vi "Actor Core.vi"(8 "error in":errorcluster, 11 "Nested in":refnum<class "GUI_Actor.lvclass">) -> (0 "error out":errorcluster, 3 "Actor out":refnum<class "Actor.lvclass">)   [LabVIEW 2019, in "GUI_Actor.lvlib" / "GUI_Actor.lvclass"]
doc: "(<B>Filename</B>: Actor Framework.lvlib:Actor.lvclass:Actor Core.vi)\n\nReceives messages to the actor, reacts to them, and initiates any error handling that may shut the actor down.\n\nDescendant classes may override this VI to append parallel tasks for the actor to complete while it handles messages. Overrides use the Call Parent Method node."
uses:
  GUI_Actor.lvclass
  C:/Program Files/National Instruments/LabVIEW 2019/vi.lib/ActorFramework/Actor/Actor.lvclass
  <vilib>/ActorFramework/Actor/Actor.lvclass
  Signal_Gen/Signal_Gen/Signal_Gen.lvclass
  Logging_txt/Logging_txt/Logging_txt.lvclass
  GUI_Actor.lvclass/GUI_Actor.ctl
  <vilib>/ActorFramework/Actor/Actor.lvclass/Actor.ctl
  <vilib>/ActorFramework/Message Enqueuer/Message Enqueuer.lvclass/Message Enqueuer.ctl
  GUI_Actor Messages/Start_Stop Msg/Start_Stop Msg.lvclass/Start_Stop Msg.ctl
  GUI_Actor Messages/Save_enable Msg/Save_enable Msg.lvclass/Save_enable Msg.ctl
  GUI_Actor Messages/File_path Msg/File_path Msg.lvclass/File_path Msg.ctl
  <vilib>/ActorFramework/Message Enqueuer/Init from Existing Queue.vi
  <vilib>/ActorFramework/Message Enqueuer/Enqueue.vi
  <vilib>/ActorFramework/Stop Msg/Stop Msg.lvclass
  C:/Program Files/National Instruments/LabVIEW 2019/vi.lib/ActorFramework/Message/Message.lvclass
  GUI_Actor Messages/Start_Stop Msg/Start_Stop Msg.lvclass
  GUI_Actor Messages/Save_enable Msg/Save_enable Msg.lvclass
  GUI_Actor Messages/File_path Msg/File_path Msg.lvclass
  <vilib>/ActorFramework/Message Priority Queue/Priority Enqueue.vi
  <vilib>/ActorFramework/Message Enqueuer/Message Enqueuer.lvclass
panel:
  out "Grafica":waveform(dbl)(graph)
  in  "Formato":enum16{"TXT", "TDMS"}(ring)
  in  "Amplitud":dbl
  in  "Frecuencia":dbl
  in  "Tipo de señal":enum16{"Senoidal", "Cuadrada", "Triangular"}(ring)
  in  "Stop":bool
  in  "Start":bool
  in  "Save":bool
  in  "Direccion":path
  in  "Exit":bool
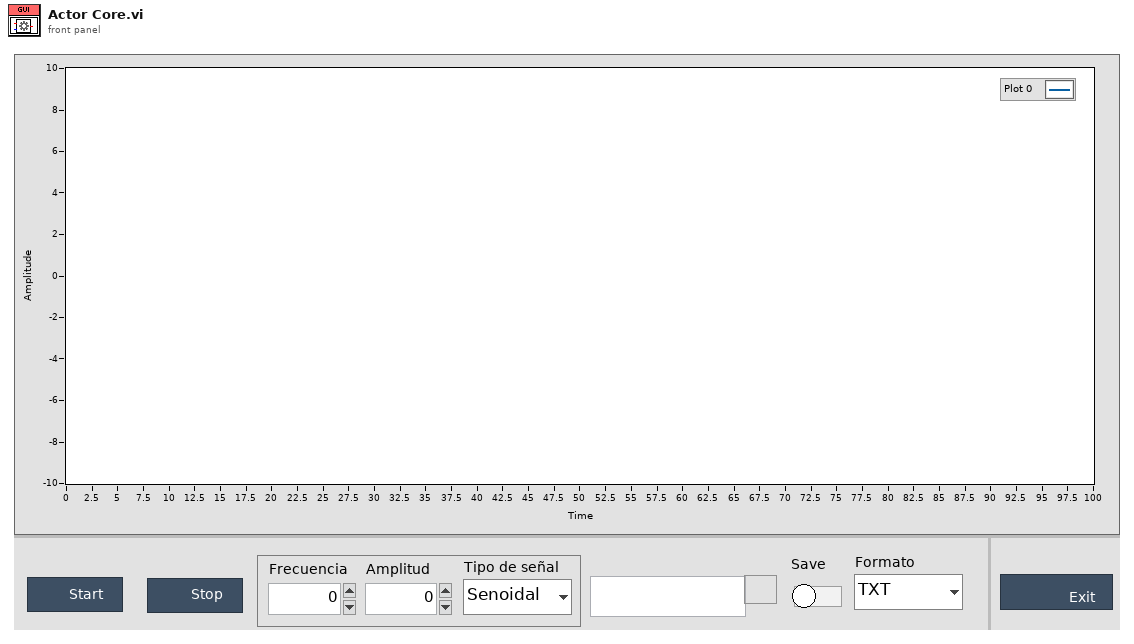
[diagram p1: front panel]
types:
  T1 = cluster{"Stop":refnum<user-event>, "Grafica":refnum<user-event>}
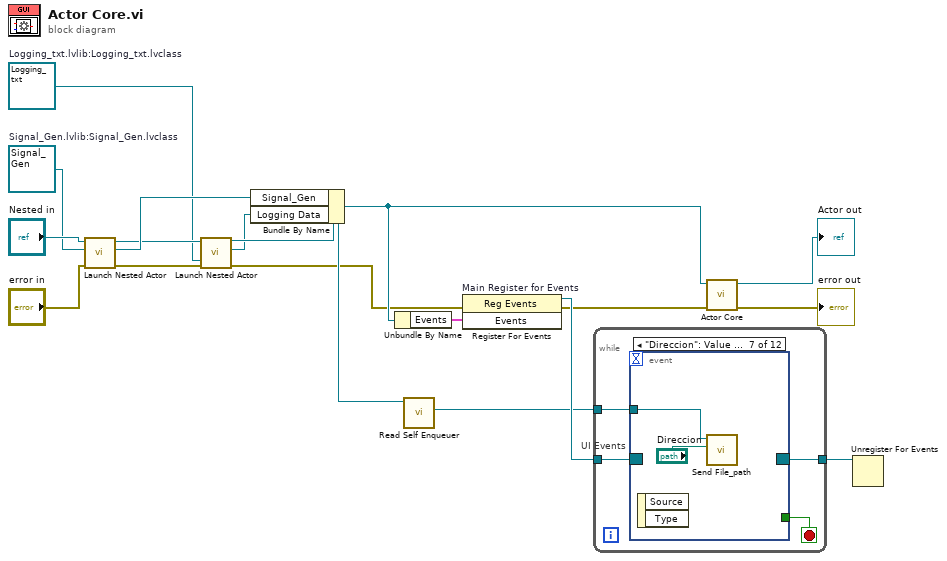
[diagram p0: block diagram]
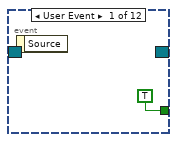
[diagram p2: hidden frame]
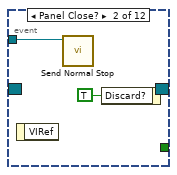
[diagram p3: hidden frame]
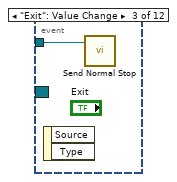
[diagram p4: hidden frame]
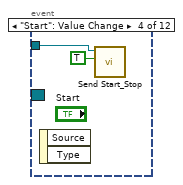
[diagram p5: hidden frame]
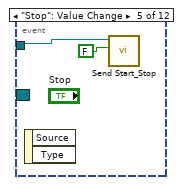
[diagram p6: hidden frame]
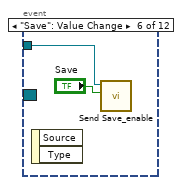
[diagram p7: hidden frame]
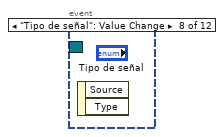
[diagram p8: hidden frame]
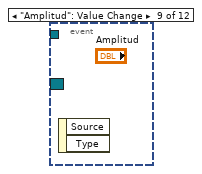
[diagram p9: hidden frame]
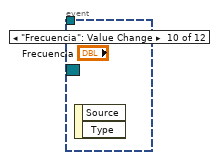
[diagram p10: hidden frame]
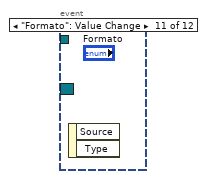
[diagram p11: hidden frame]
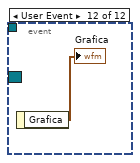
[diagram p12: hidden frame]
diagram:
  w4 = refnum<class "Logging_txt.lvclass"> refnum  # Logging_txt.lvlib:Logging_txt.lvclass
  w9 = refnum<class "Signal_Gen.lvclass"> refnum  # Signal_Gen.lvlib:Signal_Gen.lvclass
  n1 = call <vilib>:"Launch Nested Actor.vi"("error in (no error)"="error in", "Nested Actor"=w9, "Caller Actor in"="Nested in") -> ("error out"=w3:errorcluster, "Nested Actor's Enqueuer"=w7:refnum<class "Message Enqueuer.lvclass">, "Caller Actor out"=w5:refnum<class "GUI_Actor.lvclass">)  [unwired: 6 in]
  n2 = call <vilib>:"Launch Nested Actor.vi"("error in (no error)"=w3, "Nested Actor"=w4, "Caller Actor in"=w5) -> ("error out"=w2:errorcluster, "Nested Actor's Enqueuer"=w1:refnum<class "Message Enqueuer.lvclass">, "Caller Actor out"=w6:refnum<class "GUI_Actor.lvclass">)  [unwired: 6 in]
  n3 = Bundle By Name(cluster=w6, "Signal_Gen"=w7, "Logging Data"=w1) -> (w8:refnum<class "GUI_Actor.lvclass">)
  n4 = Unbundle By Name(w8) -> ("Events"=w15:T1)
  n5 = call <vilib>:"Read Self Enqueuer.vi"("Actor"=w8) -> ("Self Enqueuer"=w13:refnum<class "Message Enqueuer.lvclass">)  [unwired: 10 in]
  n6 = register-events "Main Register for Events"(error in=w2, w15) -> (reference out=w16:refnum<event-registration>, error out=w12:errorcluster)  [unwired: 1 in]
  n7 = while {
    tunnel: w16 -> [w22]
    tunnel: [w20] -> w14
    tunnel: w13 -> [w19]
    stop <- w21 stop-if-true
    n8 = event "UI Events" shown="[6] \"Direccion\": Value Change" {
      selector: w22 -> [_ _ _ _ _ _ _ _ _ _ _ _]
      dyn-events: [_ _ _ _ _ _ _ _ _ _ _ _] -> w20
      timeout: _ -> [_ _ _ _ _ _ _ _ _ _ _ _]
      tunnel: [TRUE _ _ _ _ _ _ _ _ _ _ _] -> w21
      tunnel: w19 -> [_ w24 w26 w28 w29 w32 w33 _ _ _ _ _]
      event User Event {
        n9 = event-data() -> ()  [unwired: 1 in, 1 out]
      }
      event Panel Close? {
        n10 = event-data() -> ()  [unwired: 1 in, 1 out]
        n11 = call <vilib>:"Send Normal Stop.vi"("Message Enqueuer"=w24) -> ()  [unwired: 10 in, 1 out]
        n12 = event-data("Discard?"=TRUE) -> ()  [unwired: 1 in, 1 out]
      }
      event "Exit": Value Change {
        n13 = event-data() -> ()  [unwired: 1 in, 2 out]
        n14 = call <vilib>:"Send Normal Stop.vi"("Message Enqueuer"=w26) -> ()  [unwired: 10 in, 1 out]
      }
      event "Start": Value Change {
        n15 = event-data() -> ()  [unwired: 1 in, 2 out]
        n16 = call "Send Start_Stop.vi"("Start/Stop"=TRUE, "Message Enqueuer"=w28) -> ()  [unwired: 8 in, 2 out]
      }
      event "Stop": Value Change {
        n17 = event-data() -> ()  [unwired: 1 in, 2 out]
        n18 = call "Send Start_Stop.vi"("Start/Stop"=FALSE, "Message Enqueuer"=w29) -> ()  [unwired: 8 in, 2 out]
      }
      event "Save": Value Change {
        n19 = event-data() -> ()  [unwired: 1 in, 2 out]
        n20 = call "Send Save_enable.vi"("Save?"="Save", "Message Enqueuer"=w32) -> ()  [unwired: 8 in, 2 out]
      }
      event "Direccion": Value Change {
        n21 = event-data() -> ()  [unwired: 1 in, 2 out]
        n22 = call "Send File_path.vi"("Direccion"="Direccion", "Message Enqueuer"=w33) -> ()  [unwired: 8 in, 2 out]
      }
      event "Tipo de señal": Value Change {
        n23 = event-data() -> ()  [unwired: 1 in, 2 out]
      }
      event "Amplitud": Value Change {
        n24 = event-data() -> ()  [unwired: 1 in, 2 out]
      }
      event "Frecuencia": Value Change {
        n25 = event-data() -> ()  [unwired: 1 in, 2 out]
      }
      event "Formato": Value Change {
        n26 = event-data() -> ()  [unwired: 1 in, 2 out]
      }
      event User Event {
        n27 = event-data() -> ("Grafica"=→"Grafica":waveform(dbl))  [unwired: 1 in]
      }
    }
  }
  n28 = call-parent "Actor Core.vi"("error in"=w12, "Actor in"=w8) -> ("error out"=→"error out":errorcluster, "Actor out"=→"Actor out":refnum<class "Actor.lvclass">)  [unwired: 8 in]
  n29 = Unregister For Events(event registration refnum=w14) -> ()  [unwired: 1 in, 1 out]
